vi "UI_Graph.vi"() -> ()   [LabVIEW 2016]
uses:
  PanelSplitToolkit/QueueManager.llb/Remove.vi
  PanelSplitToolkit/QueueManager.llb/Insert.vi
  PanelSplitToolkit/PanelRootNode/PanelRootNode.lvclass
  PCM PanelSplit/PCM PanelSplit.lvclass
  PanelSplitToolkit/QueueManager.llb/Destroy.vi
  <vilib>/Utility/error.llb/DialogType.ctl
  PanelSplitToolkit/QueueManager.llb/CreatQueue.vi
panel:
  in  "Caller":string
  in  "删除按钮":bool
  in  "添加按钮":bool
  in  "下一页":bool
  in  "上一页":bool
  in  "Page":u16(ring) items=["Page0"]
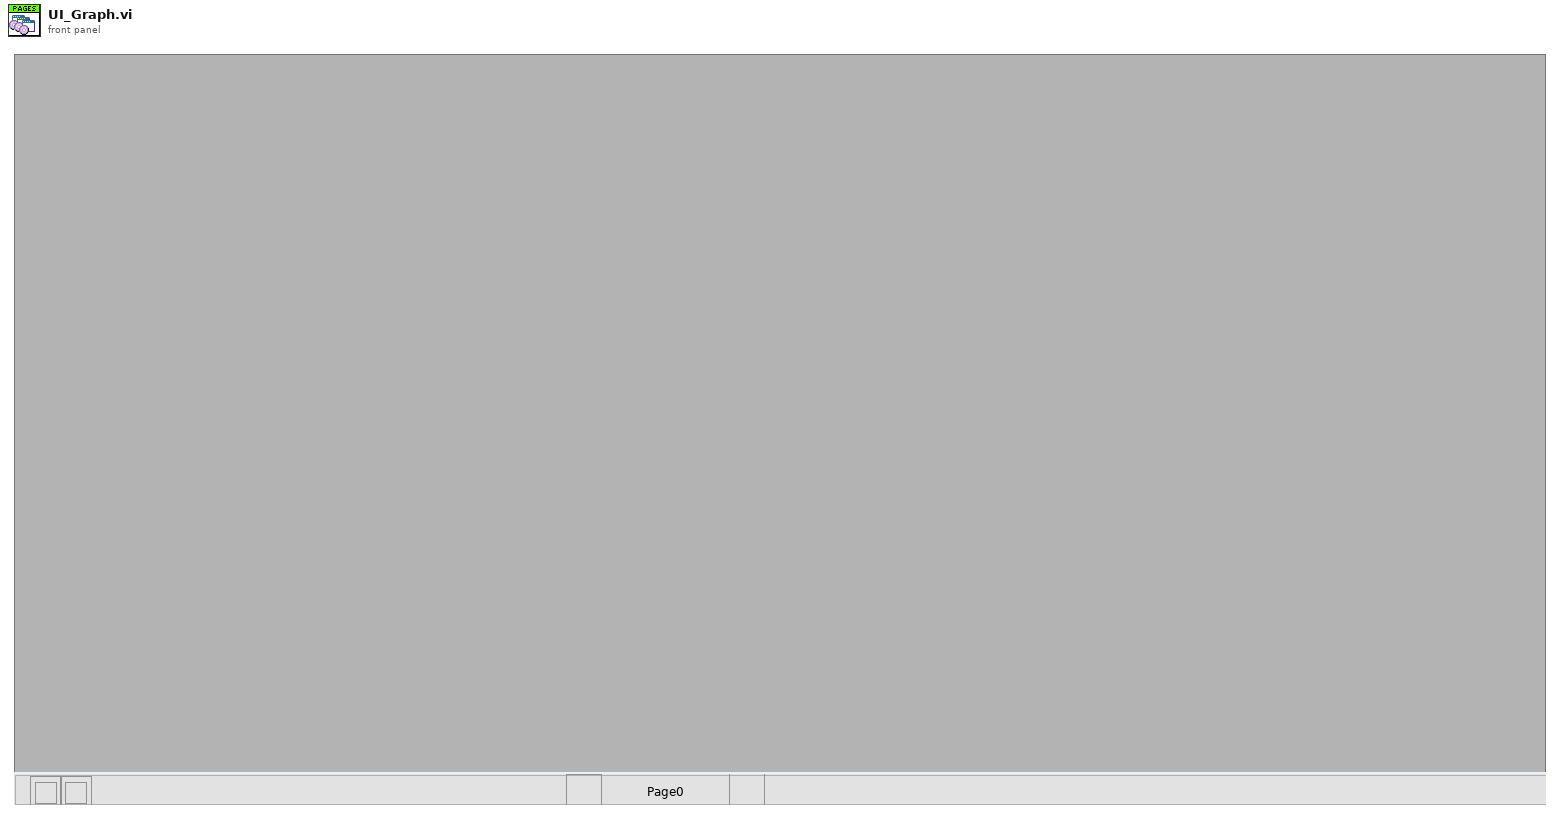
[diagram p1: front panel]
types:
  T1 = cluster{"error":errorcluster, "Event":string, "Data":variant, "Q_Local":string, "DyPageNames":string[], "DyPageVIRefs":refnum<vi>[], "PageTreeTags":string[], "CurrentPage":string, "PageVIPath":path, "PanelUIQName":string, "Send":cluster{"VI*ToSend":refnum<vi>, "EventToSend":string, "DataToSend":variant}, "PageCtr*":refnum<vi>, "SubPanel*":refnum<vi>, "Q_Caller":string, "FixedPages":cluster{"FixedPageNames":string[], "FixedPageVIRefs":refnum<vi>[]}}
  T2 = cluster{"Main Queue":string, "DAQ Queue":string, "ANA Queue":string, "CUI Queue":string, "Q-FocusList":string, "Q-Toolbar":string, "Q-Config":string}
  T3 = cluster{"Page":refnum<vi>, "SubPanel":refnum<vi>}
  T4 = typedef "DialogType.ctl" = u16
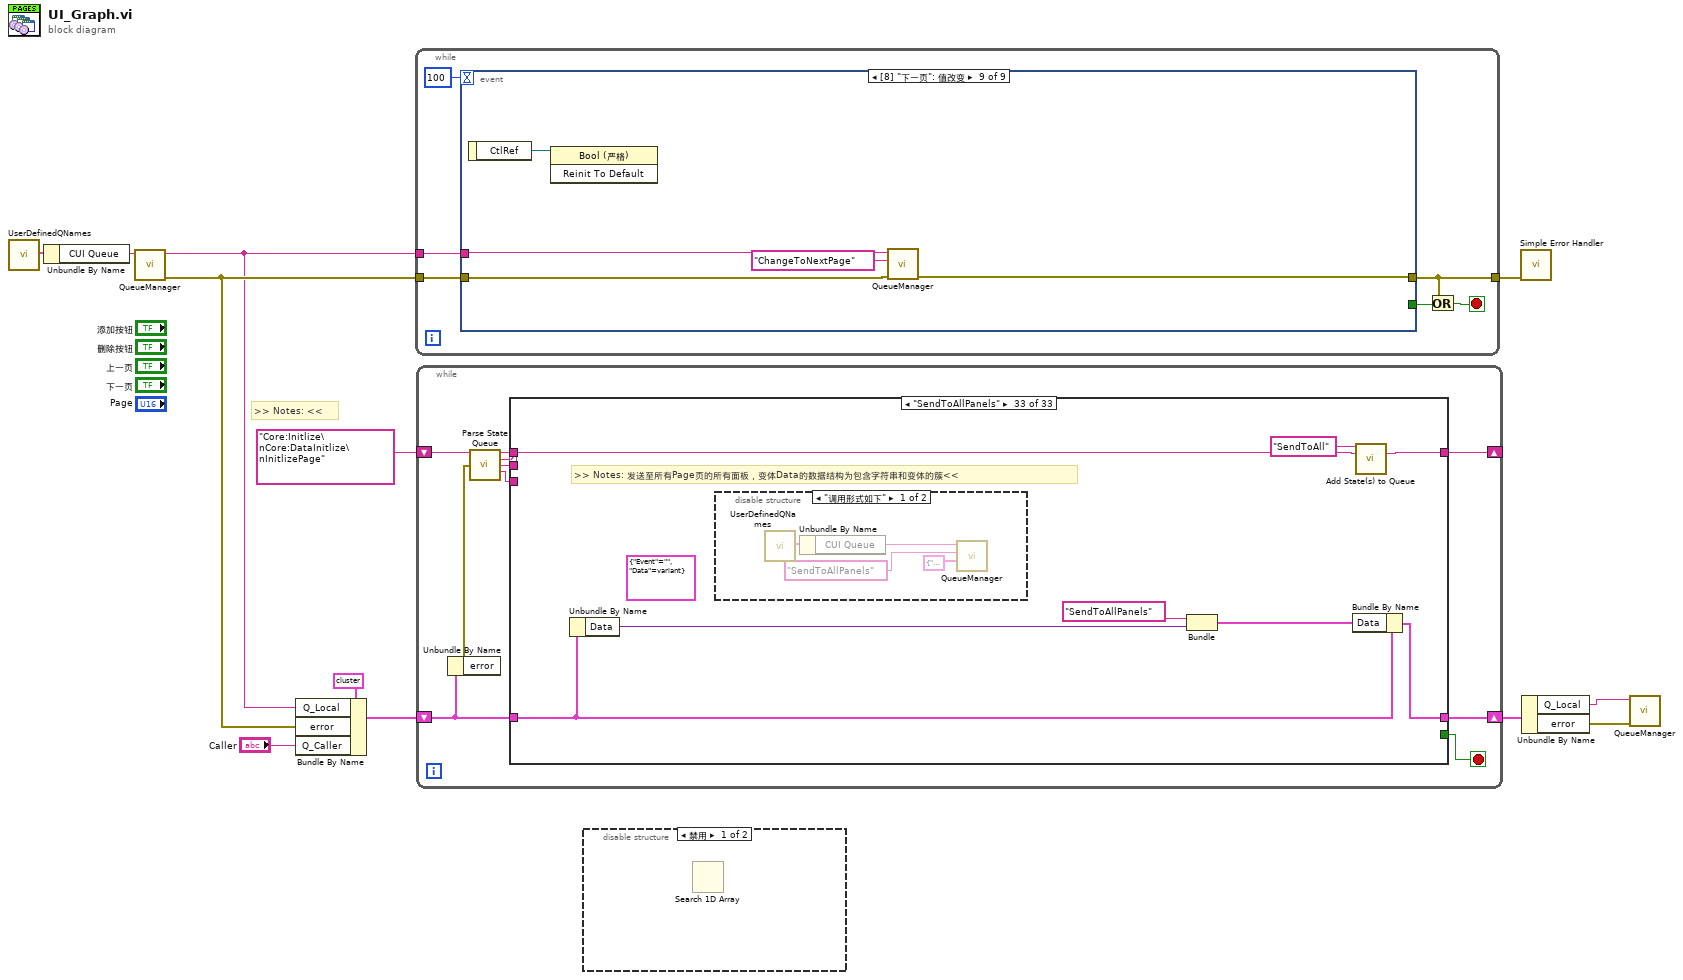
[diagram p0: block diagram]
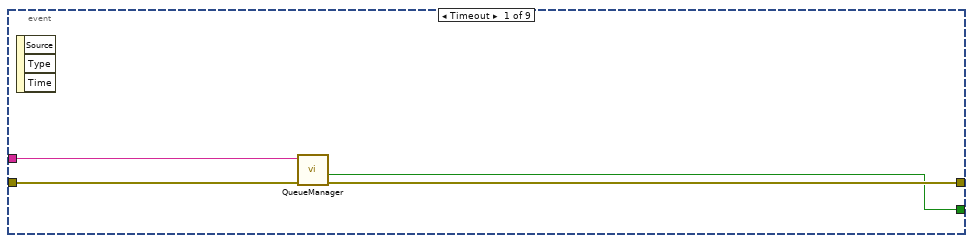
[diagram p2: hidden frame]
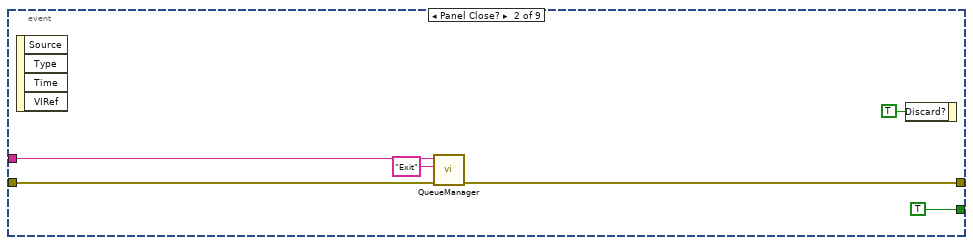
[diagram p3: hidden frame]
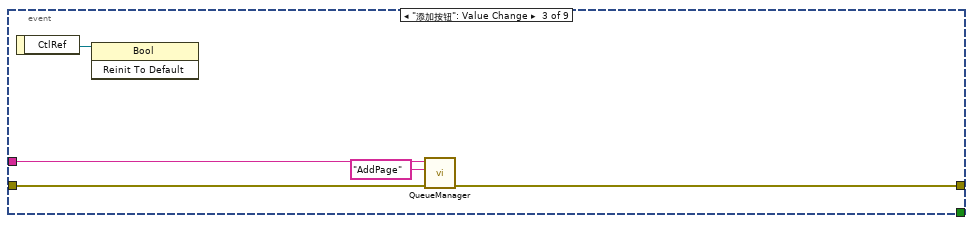
[diagram p4: hidden frame]
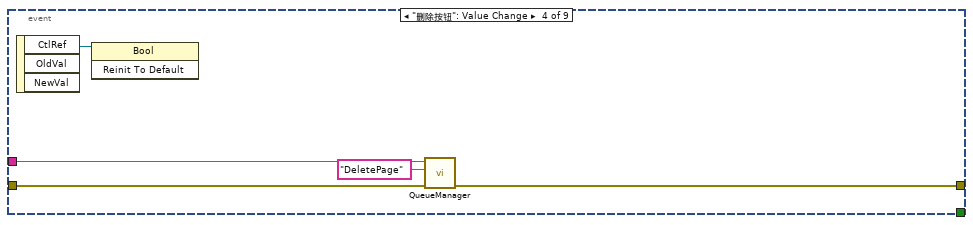
[diagram p5: hidden frame]
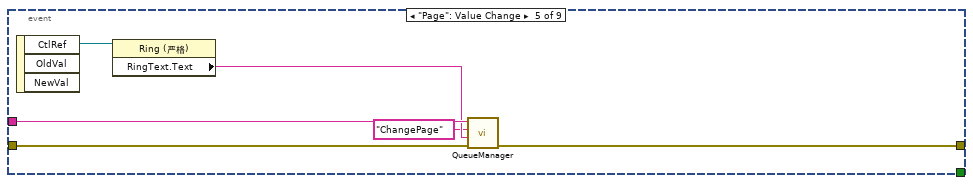
[diagram p6: hidden frame]
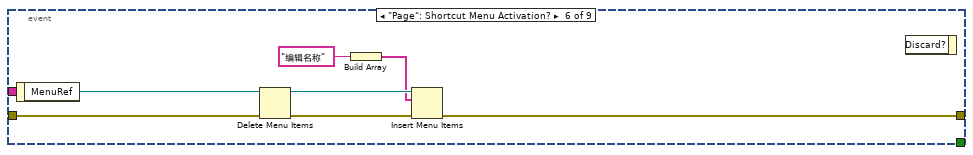
[diagram p7: hidden frame]
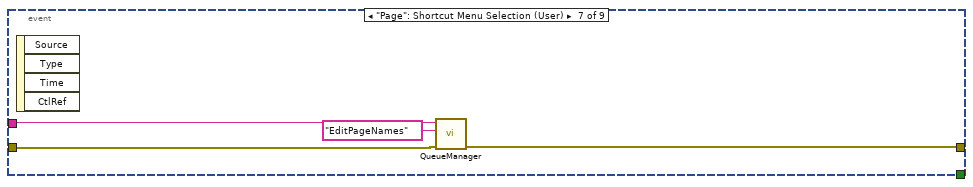
[diagram p8: hidden frame]
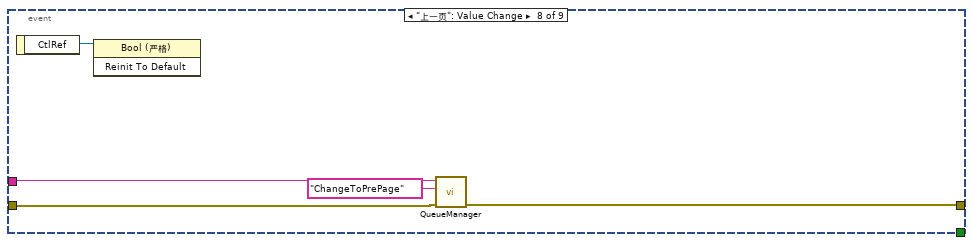
[diagram p9: hidden frame]
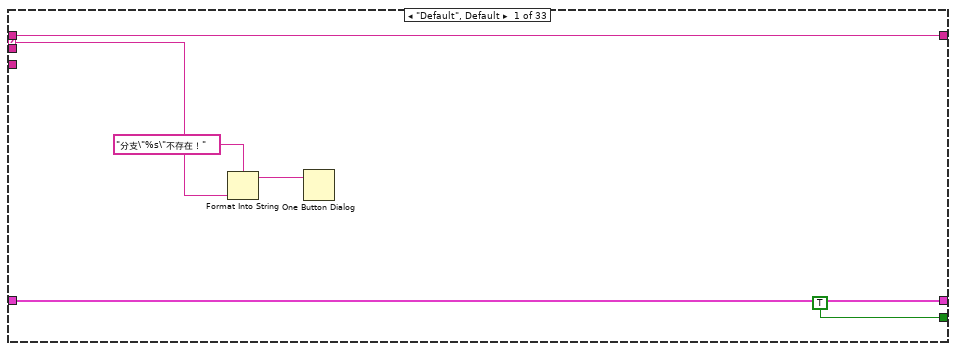
[diagram p11: hidden frame]
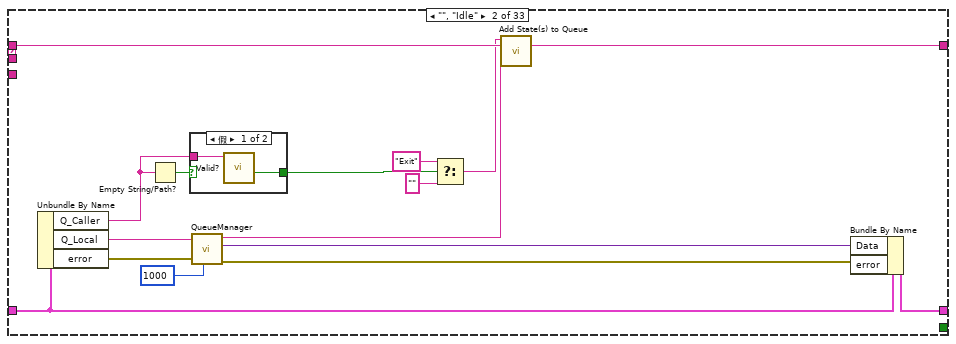
[diagram p12: hidden frame]
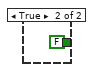
[diagram p13: hidden frame]
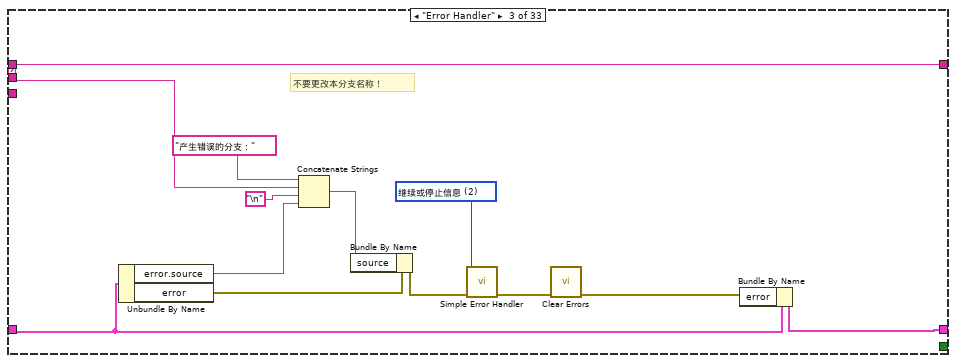
[diagram p14: hidden frame]
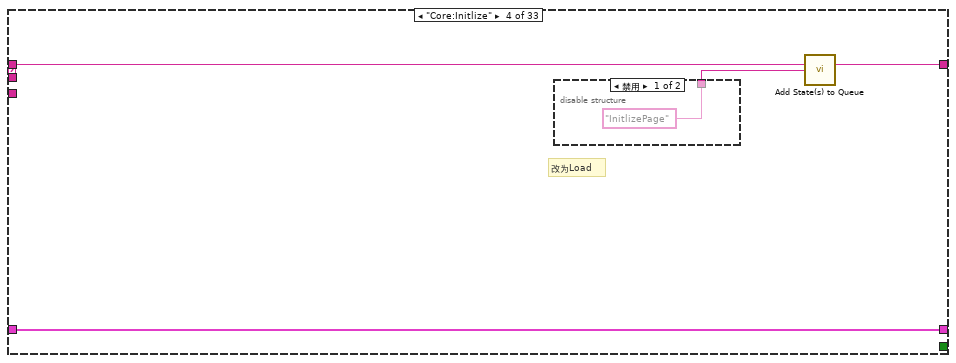
[diagram p15: hidden frame]
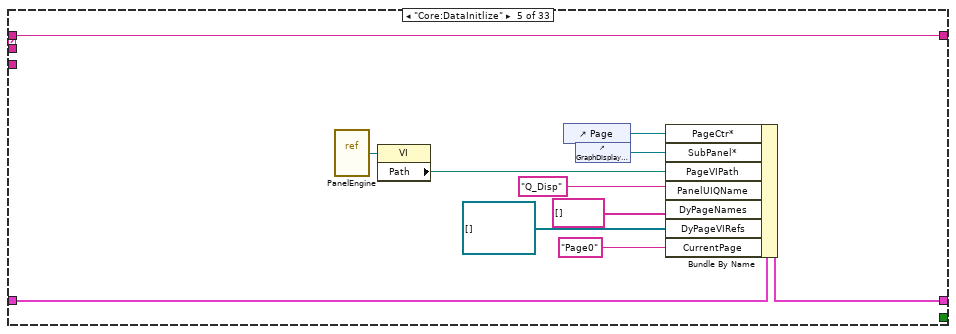
[diagram p17: hidden frame]
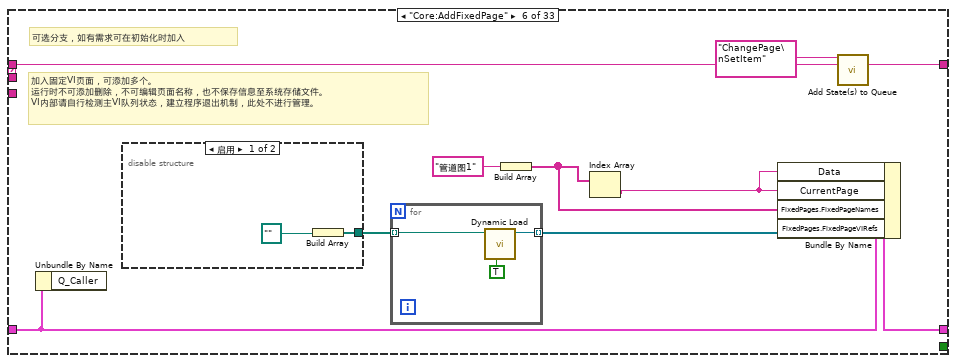
[diagram p18: hidden frame]
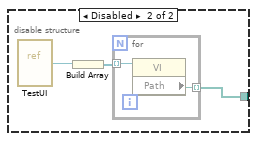
[diagram p19: hidden frame]
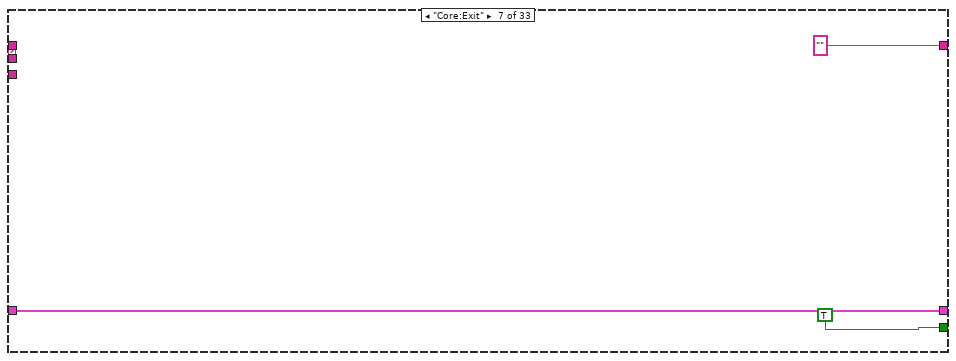
[diagram p20: hidden frame]
diagram:
  # ">> Notes: <<"
  n1 = call "UserDefinedQNames.vi"() -> ("All Queues"=w2:T2)  [unwired: 11 in]
  n2 = Unbundle By Name(w2) -> ("CUI Queue"=w1:string)
  n3 = call-poly "QueueManager.vi"("QueueName"=w1) -> ("error out"=w6:errorcluster, "QueueName out"=w4:string)  [unwired: 9 in]
  n4 = Bundle By Name(cluster=T1 {"error"={"status"=FALSE, "code"=0, "source"=""}, "Event"="", "Data"=variant, "Q_Local"="", "DyPageNames"=[], "DyPageVIRefs"=[], "PageTreeTags"=[], "CurrentPage"="", "PageVIPath"=path "", "PanelUIQName"="", "Send"={"VI*ToSend"=refnum, "EventToSend"="", "DataToSend"=variant}, "PageCtr*"=refnum, "SubPanel*"=refnum, "Q_Caller"="", "FixedPages"={"FixedPageNames"=[], "FixedPageVIRefs"=[]}} ("TmpData"), "Q_Local"=w4, "error"=w6, "Q_Caller"="Caller") -> (w8:T1)
  n5 = while {
    tunnel: w6 -> [w17]
    tunnel: [w15] -> w5
    tunnel: w4 -> [w13]
    stop <- w18 stop-if-true
    n6 = event shown="[8] \"下一页\": 值改变" {
      selector: _ -> [_ _ _ _ _ _ _ _ _]
      dyn-events: _ -> [_ _ _ _ _ _ _ _ _]
      timeout: 100 -> [_ _ _ _ _ _ _ _ _]
      tunnel: w17 -> [w21 w26 w31 w36 w42 w46 w55 w60 w65]
      tunnel: [w20 w25 w30 w35 w41 w45 w52 w57 w62] -> w15
      tunnel: [w19 TRUE _ _ _ _ _ _ _] -> w16
      tunnel: w13 -> [w22 w27 w32 w37 w43 _ w54 w59 w64]
      event Timeout {
        n7 = event-data() -> ()  [unwired: 1 in, 3 out]
        n8 = call-poly "QueueManager.vi"("error in (no error)"=w21, "Queue Name(unamed)"=w22) -> ("error out"=w20:errorcluster, "Not Exist?"=w19:bool)  [unwired: 8 in]
      }
      event Panel Close? {
        n9 = event-data() -> ()  [unwired: 1 in, 4 out]
        n10 = call-poly "QueueManager.vi"("error in"=w26, "Event"="Exit", "QueueName"=w27) -> ("error out"=w25:errorcluster)  [unwired: 7 in, 1 out]
        n11 = event-data("Discard?"=TRUE ("放弃？")) -> ()  [unwired: 1 in, 1 out]
      }
      event "添加按钮": Value Change {
        n12 = event-data() -> ("CtlRef"=w33:refnum<vi>)  [unwired: 1 in]
        n13 = invoke class="Bool" method="Reinit To Default"(reference=w33) -> ()  [unwired: 2 in, 3 out]
        n14 = call-poly "QueueManager.vi"("error in"=w31, "Event"="AddPage", "QueueName"=w32) -> ("error out"=w30:errorcluster)  [unwired: 7 in, 1 out]
      }
      event "删除按钮": Value Change {
        n15 = event-data() -> ("CtlRef"=w38:refnum<vi>)  [unwired: 1 in, 2 out]
        n16 = invoke class="Bool" method="Reinit To Default"(reference=w38) -> ()  [unwired: 2 in, 3 out]
        n17 = call-poly "QueueManager.vi"("error in"=w36, "Event"="DeletePage", "QueueName"=w37) -> ("error out"=w35:errorcluster)  [unwired: 7 in, 1 out]
      }
      event "Page": Value Change {
        n18 = event-data() -> ("CtlRef"=w44:refnum<vi>)  [unwired: 1 in, 2 out]
        n19 = property class="Ring (严格)"(reference=w44) -> ("RingText.Text"=w40:string)  [unwired: 1 in, 2 out]
        n20 = call-poly "QueueManager.vi"("error in"=w42, "Data"=w40, "Event"="ChangePage", "QueueName"=w43) -> ("error out"=w41:errorcluster)  [unwired: 6 in, 1 out]
      }
      event "Page": Shortcut Menu Activation? {
        n21 = event-data() -> ("MenuRef"=w47:refnum<k9>)  [unwired: 1 in]
        n22 = Delete Menu Items(6:w46, 9:w47) -> (0:w50:errorcluster, 3:w51:refnum<k9>)  [unwired: 2 in]
        n23 = Build Array("编辑名称") -> (w48:string[])
        n24 = Insert Menu Items(6:w50, 8:w48, 9:w51) -> (0:w45:errorcluster)  [unwired: 3 in, 2 out]
        n25 = event-data() -> ()  [unwired: 2 in, 1 out]
      }
      event "Page": Shortcut Menu Selection (User) {
        n26 = event-data() -> ()  [unwired: 1 in, 4 out]
        n27 = call-poly "QueueManager.vi"("error in"=w55, "Event"="EditPageNames", "QueueName"=w54) -> ("error out"=w52:errorcluster)  [unwired: 7 in, 1 out]
      }
      event "上一页": Value Change {
        n28 = event-data() -> ("CtlRef"=w56:refnum<vi>)  [unwired: 1 in]
        n29 = invoke class="Bool (严格)" method="Reinit To Default"(reference=w56) -> ()  [unwired: 2 in, 3 out]
        n30 = call-poly "QueueManager.vi"("error in"=w60, "Event"="ChangeToPrePage", "QueueName"=w59) -> ("error out"=w57:errorcluster)  [unwired: 7 in, 1 out]
      }
      event "下一页": Value Change {
        n31 = event-data() -> ("CtlRef"=w61:refnum<vi>)  [unwired: 1 in]
        n32 = invoke class="Bool (严格)" method="Reinit To Default"(reference=w61) -> ()  [unwired: 2 in, 3 out]
        n33 = call-poly "QueueManager.vi"("error in"=w65, "Event"="ChangeToNextPage", "QueueName"=w64) -> ("error out"=w62:errorcluster)  [unwired: 7 in, 1 out]
      }
    }
    n34 = Or(x=w15, y=w16) -> (x .or. y?=w18:bool)
  }
  n35 = while {
    shift-right: [w68] -> w10
    shift-left: w8 -> [w69]
    shift-right: [w67] -> _
    shift-left: "Core:Initlize\nCore:DataInitlize\nInitlizePage" -> [w75]
    stop <- w71 stop-if-true
    n36 = Unbundle By Name(w69) -> ("error"=w70:errorcluster)
    n37 = call "Parse State Queue.vi"("State Queue"=w75, "Error In (no error)"=w70) -> ("Remaining States"=w74:string, "Current State"=w73:string, "Arguments"=w72:string, "PreState"=w66:string)  [unwired: 10 in]
    n38 = case shown="\"SendToAllPanels\"" w73 {
      selector: w73 -> [w79 _ _ _ _ _ _ _ _ _ _ _ _ _ _ _ _ _ _ _ _ _ _ _ _ _ _ _ _ _ _ _ _]
      tunnel: w74 -> [w80 w93 w113 w116 w129 w133 _ _ w158 w166 w168 w194 w219 w242 w257 w276 w278 w283 w304 w332 w336 w345 w403 w408 w433 w446 w457 w468 w472 w493 w495 w507 w517]
      tunnel: w72 -> [_ _ w101 _ _ _ _ _ _ _ _ _ _ _ _ _ _ _ _ _ _ _ _ _ _ _ _ _ _ _ _ _ _]
      tunnel: [TRUE _ _ _ _ _ TRUE FALSE FALSE _ _ _ _ _ _ _ FALSE FALSE _ _ _ _ _ _ _ _ _ _ _ _ _ _ _] -> w71
      tunnel: w69 -> [w81 w90 w103 w117 w128 w131 w151 w154 w162 w165 w176 w192 w209 w240 w261 w277 w279 w284 w313 w327 w338 w347 w395 w410 w435 w445 w448 w459 w477 w488 w494 w498 w519]
      tunnel: [w81 w96 w102 w117 w127 w139 w151 w153 w161 w165 w175 w191 w207 w239 w260 w277 w279 w285 w311 w326 w337 w346 w394 w409 w434 w445 w447 w458 w473 w486 w494 w497 w514] -> w68
      tunnel: [w80 w92 w113 w115 w129 w132 "" ("Remaining States") "SendToAll\nCore:Exit" ("Remaining States") w159 w166 w167 w194 w218 w241 w256 w275 w278 w282 w303 w332 w335 w344 w403 w407 w432 w446 w457 w468 w471 w493 w495 w507 w516] -> w67
      tunnel: w66 -> [_ _ _ _ _ _ _ _ _ _ _ _ _ _ _ _ _ _ _ _ _ _ _ _ _ _ _ _ _ _ _ _ _]
      frame "Default", Default {
        n39 = Format Into String(format string="分支\"%s\"不存在！" ("格式字符串"), w79) -> (resulting string=w78:string)  [unwired: 2 in, 1 out]
        n40 = One Button Dialog(message=w78) -> ()  [unwired: 1 in, 1 out]
      }
      frame "", "Idle" {
        n41 = Unbundle By Name(w90) -> ("Q_Caller"=w83:string, "Q_Local"=w89:string, "error"=w88:errorcluster)
        n42 = Empty String/Path?(string/path=w83) -> (empty?=w87:bool)
        n43 = case shown="假" w87 {
          tunnel: [w99 FALSE ("Not Exist?")] -> w86
          tunnel: w83 -> [w98 _]
          frame False {
            n44 = call "Valid?.vi"("Queue Name(unamed)"=w98) -> ("Not Exist?"=w99:bool)  [unwired: 9 in, 1 out]
          }
          frame True {
          }
        }
        n45 = call-poly "QueueManager.vi"("Time out(-1)"=1000, "error in (no error)"=w88, "Queue Name"=w89) -> ("error out"=w97:errorcluster, "Data"=w95:variant, "Event"=w94:string)  [unwired: 5 in, 1 out]
        n46 = Select(t="Exit" ("Event"), s=w86, f="") -> (s? t:f=w82:string)
        n47 = call "Add State(s) to Queue.vi"("State(s) in Front (\"\")"=w82, "State(s) in (\"\")"=w93, "State(s) at Back (\"\")"=w94) -> ("States Out"=w92:string)  [unwired: 12 in]
        n48 = Bundle By Name(cluster=w90, "Data"=w95, "error"=w97) -> (w96:T1)
      }
      frame "Error Handler" {
        w110 = T4 2 items=["无对话框", "确定信息", "继续或停止信息", "确定信息＋警告", "继续/停止+警告"] ("type of dialog (OK msg:1)")
        # "不要更改本分支名称！"
        n49 = Unbundle By Name(w103) -> ("error.source"=w104:string, "error"=w106:errorcluster)
        n50 = Concatenate Strings("产生错误的分支：" ("字符串"), w101, "\n", w104) -> (w107:string)
        n51 = Bundle By Name(cluster=w106, "source"=w107) -> (w105:errorcluster)
        n52 = call <vilib>:"Simple Error Handler.vi"("type of dialog (OK msg:1)"=w110, "error in (no error)"=w105) -> ("error out"=w111:errorcluster)  [unwired: 3 in, 4 out]
        n53 = call <vilib>:"Clear Errors.vi"("error in (no error)"=w111) -> ("error out"=w112:errorcluster)  [unwired: 5 in, 1 out]
        n54 = Bundle By Name(cluster=w103, "error"=w112) -> (w102:T1)
      }
      frame "Core:Initlize" {
        # "改为Load"
        n55 = disable-structure shown="禁用" {
          disable-tunnel: ["InitlizePage" ("State(s) at Back (\"\")") _] -> w114
          frame Disabled {
          }
          frame Enabled {
          }
        }
        n56 = call "Add State(s) to Queue.vi"("State(s) in (\"\")"=w116, "State(s) at Back (\"\")"=w114) -> ("States Out"=w115:string)  [unwired: 13 in]
      }
      frame "Core:DataInitlize" {
        n57 = vi-ref "PanelEngine.vi"() -> (w125:refnum<vi>)
        n58 = property class="VI"(reference=w125) -> ("Path"=w124:path)  [unwired: 1 in, 2 out]
        n59 = control-ref of="Page"() -> (w120:refnum<vi>)
        n60 = control-ref of="GraphDisplayPanel"() -> (w119:refnum<vi>)
        n61 = Bundle By Name(cluster=w128, "PageCtr*"=w120, "SubPanel*"=w119, "PageVIPath"=w124, "PanelUIQName"="Q_Disp", "DyPageNames"=string[] [] ("PageNames"), "DyPageVIRefs"=refnum<vi>[] [] ("PageVIRefs"), "CurrentPage"="Page0") -> (w127:T1)
      }
      frame "Core:AddFixedPage" {
        # "可选分支，如有需求可在初始化时加入"
        # "加入固定VI页面，可添加多个。\n运行时不可添加删除，不可编辑页面名称，也不保存信息至系统存储文件。\nVI内部请自行检测主VI队列状态，建立程序退出机制，此处不进行管理。"
        n62 = Unbundle By Name(w131) -> ()  [unwired: 1 out]
        n63 = disable-structure shown="启用" {
          disable-tunnel: [w140 w144] -> w137
          frame Enabled {
            n64 = Build Array(path "" ("Vi Path")) -> (w140:path[])
          }
          frame Disabled {
            n65 = vi-ref "TestUI.vi"() -> (w142:refnum<vi>)
            n66 = Build Array(w142) -> (w143:refnum<vi>[])
            n67 = for {
              tunnel: w143 -> [w146] mode=indexing
              tunnel: [w145] -> w144 mode=indexing
              n68 = property class="VI"(reference=w146) -> ("Path"=w145:path)  [unwired: 1 in, 2 out]
            }
          }
        }
        n69 = for {
          tunnel: [w149] -> w138 mode=indexing
          tunnel: w137 -> [w148] mode=indexing
          n70 = call "Dynamic Load.vi"("Auto Dispose Ref"=TRUE, "Vi Path"=w148) -> ("vi reference"=w149:refnum<vi>)  [unwired: 8 in, 1 out]
        }
        n71 = Build Array("管道图1") -> (w135:string[])
        n72 = Index Array(array=w135) -> (element=w130:string)  [unwired: 1 in]
        n73 = Bundle By Name(cluster=w131, "Data"=w130, "CurrentPage"=w130, "FixedPages.FixedPageNames"=w135, "FixedPages.FixedPageVIRefs"=w138) -> (w139:T1)
        n74 = call "Add State(s) to Queue.vi"("State(s) in Front (\"\")"="ChangePage\nSetItem" ("State(s) in Front (\"\")"), "State(s) in (\"\")"=w133) -> ("States Out"=w132:string)  [unwired: 13 in]
      }
      frame "Core:Exit" {
      }
      frame "Exit" {
        n75 = Bundle By Name(cluster=w154, "Data"=cluster{string, "变体":variant} {"Exit", "变体"=variant}) -> (w153:T1)
      }
      frame "Clear" {
        n76 = Bundle By Name(cluster=w162, "Data"=cluster{string, "变体":variant} {"Exit", "变体"=variant}) -> (w161:T1)
        n77 = call "Add State(s) to Queue.vi"("State(s) in Front (\"\")"="SendToAll\nCore:DataInitlize" ("Remaining States"), "State(s) in (\"\")"=w158) -> ("States Out"=w159:string)  [unwired: 13 in]
      }
      frame "--------Init------------" {
      }
      frame "Initlize" {
        n78 = Unbundle By Name(w176) -> ("Data"=w178:variant, "error"=w170:errorcluster)
        n79 = Variant To Data(error in=w170, type=T3 {"Page"=refnum, "SubPanel"=refnum}, Variant=w178) -> (data=w174:T3, error out=w171:errorcluster)
        n80 = Unbundle By Name(w174) -> ("Page"=w173:refnum<vi>, "SubPanel"=w172:refnum<vi>)
        n81 = Bundle By Name(cluster=w176, "PageCtr*"=w173, "SubPanel*"=w172, "error"=w171) -> (w175:T1)
        n82 = call "Add State(s) to Queue.vi"("State(s) in (\"\")"=w168, "State(s) at Back (\"\")"="InitlizePage" ("State(s) in Front (\"\")")) -> ("States Out"=w167:string)  [unwired: 13 in]
      }
      frame "Save" {
        w189 = ""  # Q_Name
        # ">> Notes: 获取所有Page页的保存信息，发送给请求保存的队列<<"
        n83 = Unbundle By Name(w192) -> ("DyPageNames"=w180:string[], "DyPageVIRefs"=w193:refnum<vi>[], "Data"=w190:variant, "error"=w183:errorcluster)
        n84 = Variant To Data(error in=w183, type=w189, Variant=w190) -> (data=w186:string, error out=w184:errorcluster)
        n85 = for {
          tunnel: w193 -> [w198] mode=indexing
          tunnel: [w200] -> w182 mode=indexing
          shift-right: [w199] -> w188
          shift-left: w184 -> [w195]
          n86 = call "Get RootNodebyVIRef.vi"("error in"=w195, "vi*"=w198) -> ("error out"=w196:errorcluster, "RootNode*"=w197:refnum<data-value>)  [unwired: 8 in]
          n87 = in-place {
            in-place-border: w196 -> [w203]
            in-place-border: [w202] -> w199
            in-place-border: [w201] -> w200
            n88 = in-place-dvr #1(w197) -> (w205:refnum<class "PanelRootNode.lvclass">)  [unwired: 1 out]
            n89 = call-dynamic "GetXmlString.vi"("error in"=w203, "PanelRootNode 输入"=w205) -> ("error out"=w202:errorcluster, "XML"=w201:string, "PanelRootNode 输出"=w204:refnum<class "PanelRootNode.lvclass">)  [unwired: 7 in]
            n90 = in-place-dvr #1(w204) -> ()  [unwired: 2 out]
          }
        }
        n91 = Flatten To XML(anything=w180) -> (xml string=w179:string)
        n92 = Build Array (concatenate)(w179, w182) -> (w181:string[])
        n93 = call-poly "QueueManager.vi"("error in"=w188, "Data"=w181, "Event"="Save", "QueueName"=w186) -> ("error out"=w187:errorcluster)  [unwired: 6 in, 1 out]
        n94 = Bundle By Name(cluster=w192, "error"=w187) -> (w191:T1)
      }
      frame "Load11" {
        # ">> Notes: 装载配置信息\n1.清除当前所有图和页面\n2.根据配置信息增加相应页\n3.每个页读取配置文件进行分割及节点赋值<<"
        n95 = Unbundle By Name(w209) -> ("Q_Local"=w211:string, "Data"=w216:variant)
        n96 = call-poly "QueueManager.vi"("Event"="Clear", "QueueName"=w211) -> ("error out"=w214:errorcluster)  [unwired: 8 in, 1 out]
        n97 = Variant To Data(error in=w214, type=string[] [], Variant=w216) -> (data=w206:string[], error out=w213:errorcluster)
        n98 = for {
          tunnel: w211 -> [w222]
          tunnel: w206 -> [_] mode=indexing
          shift-right: [w220] -> w212
          shift-left: w213 -> [w223]
          n99 = call-poly "QueueManager.vi"("error in"=w223, "Event"="AddPage", "QueueName"=w222) -> ("error out"=w220:errorcluster)  [unwired: 7 in, 1 out]
        }
        n100 = call-poly "QueueManager.vi"("error in"=w212, "Data"=w206, "Event"="LoadXml", "QueueName"=w211) -> ("error out"=w208:errorcluster)  [unwired: 6 in, 1 out]
        n101 = call "Add State(s) to Queue.vi"("State(s) in (\"\")"=w219) -> ("States Out"=w218:string)  [unwired: 14 in]
        n102 = Bundle By Name(cluster=w209, "error"=w208) -> (w207:T1)
      }
      frame "Load" {
        # ">> Notes: 装载配置信息\n1.清除当前所有图和页面\n2.根据配置信息增加相应页\n3.每个页读取配置文件进行分割及节点赋值<<"
        n103 = Unbundle By Name(w240) -> ("SubPanel*"=w231:refnum<vi>, "PageVIPath"=w232:path, "Data"=w235:variant, "DyPageVIRefs"=w238:refnum<vi>[], "error"=w237:errorcluster, "FixedPages.FixedPageNames"=w226:string[])
        n104 = for {
          tunnel: w238 -> [w250] mode=indexing
          shift-right: [w248] -> w236
          shift-left: w237 -> [w247]
          n105 = call "GetViName.vi"("VI*"=w250) -> ("VI Name"=w249:string)  [unwired: 9 in, 1 out]
          n106 = call-poly "QueueManager.vi"("error in"=w247, "Event"="Exit", "QueueName"=w249) -> ("error out"=w248:errorcluster)  [unwired: 7 in, 1 out]
        }
        n107 = Index Array(array=w226) -> (element=w225:string)  [unwired: 1 in]
        n108 = Variant To Data(error in=w236, Variant=w235) -> (data=w233:string[], error out=w234:errorcluster)  [unwired: 1 in]
        n109 = call "PageLoad.vi"("error in"=w234, "SubPanel*"=w231, "PanelVIPath"=w232, "data"=w233) -> ("error out"=w224:errorcluster, "PageNames"=w229:string[], "VIRefs"=w230:refnum<vi>[])  [unwired: 5 in]
        n110 = disable-structure shown="启用" {
          disable-tunnel: w229 -> [w244 _]
          disable-tunnel: [w243 w245] -> w228
          disable-tunnel: w225 -> [_ w245]
          frame Enabled {
            n111 = Index Array(array=w244) -> (element=w243:string)  [unwired: 1 in]
          }
          frame Disabled {
          }
        }
        n112 = call "Add State(s) to Queue.vi"("State(s) in Front (\"\")"="ChangePage\nSetItem" ("State(s) in Front (\"\")"), "State(s) in (\"\")"=w242) -> ("States Out"=w241:string)  [unwired: 13 in]
        n113 = Bundle By Name(cluster=w240, "DyPageVIRefs"=w230, "DyPageNames"=w229, "error"=w224, "Data"=w228) -> (w239:T1)
      }
      frame "LoadXml" {
        n114 = Unbundle By Name(w261) -> ("DyPageVIRefs"=w262:refnum<vi>[], "Data"=w255:variant, "error"=w251:errorcluster)
        n115 = Variant To Data(error in=w251, type=string[] [], Variant=w255) -> (data=w254:string[], error out=w252:errorcluster)
        n116 = for {
          tunnel: w262 -> [w273] mode=indexing
          tunnel: w254 -> [w272] mode=indexing
          tunnel: [w269] -> w259 mode=indexing
          tunnel: w252 -> [w263]
          n117 = call "GetViName.vi"("VI*"=w273) -> ("VI Name"=w268:string)  [unwired: 9 in, 1 out]
          n118 = call-poly "QueueManager.vi"("error in"=w263, "Data"=w272, "Event"="LoadXmlString", "QueueName"=w268) -> ("error out"=w270:errorcluster)  [unwired: 6 in, 1 out]
          n119 = Bundle By Name(cluster=cluster{"Event":string, "Data":variant} {"Event"="", "Data"=variant} ("Send"), "Event"="Load") -> (w265:cluster{"Event":string, "Data":variant})
          n120 = call-poly "QueueManager.vi"("error in"=w270, "Data"=w265, "Event"="SendToAllPanels", "QueueName"=w268) -> ("error out"=w269:errorcluster)  [unwired: 6 in, 1 out]
        }
        n121 = Merge Errors(w259) -> (w258:errorcluster)
        n122 = call "Add State(s) to Queue.vi"("State(s) in (\"\")"=w257) -> ("States Out"=w256:string)  [unwired: 14 in]
        n123 = Bundle By Name(cluster=w261, "error"=w258) -> (w260:T1)
      }
      frame "New" {
        # ">> Notes: 响应主程序的“新建”指令，清除所有页面，然后加载一个波形图表<<"
        n124 = call "Add State(s) to Queue.vi"("State(s) in (\"\")"=w276, "State(s) at Back (\"\")"="Clear\nAddPage" ("State(s) at Back (\"\")")) -> ("States Out"=w275:string)  [unwired: 13 in]
      }
      frame "-----PageManager------" {
      }
      frame "InitlizePage" {
        n125 = disable-structure shown="启用" {
          disable-tunnel: [w297 w298] -> w285
          disable-tunnel: w284 -> [w296 w298]
          disable-tunnel: ["ChangePage" ("State(s) in Front (\"\")") "AddPage" ("State(s) in Front (\"\")")] -> w281
          frame Disabled {
            w289 = "Page0" ("CurrentPage")
            n126 = Unbundle By Name(w296) -> ("PageVIPath"=w295:path, "error"=w293:errorcluster)
            n127 = call "Dynamic Load.vi"("Auto Dispose Ref"=TRUE ("自动销毁引用"), "error in"=w293, "Vi Path"=w295) -> ("错误输出"=w290:errorcluster, "vi reference"=w294:refnum<vi>)  [unwired: 7 in]
            n128 = Build Array(w294) -> (w292:refnum<vi>[])
            n129 = Build Array(w289) -> (w291:string[])
            n130 = Bundle By Name(cluster=w296, "CurrentPage"=w289, "DyPageNames"=w291, "DyPageVIRefs"=w292, "error"=w290, "Data"=w289) -> (w297:T1)
          }
          frame Enabled {
          }
        }
        n131 = call "Add State(s) to Queue.vi"("State(s) in Front (\"\")"=w281, "State(s) in (\"\")"=w283) -> ("States Out"=w282:string)  [unwired: 13 in]
      }
      frame "AddPage" {
        n132 = Unbundle By Name(w313) -> ("DyPageVIRefs"=w309:refnum<vi>[], "PageVIPath"=w310:path, "DyPageNames"=w301:string[])
        n133 = for {
          N: 100 -> [_]
          tunnel: w301 -> [w319]
          tunnel: "Page" -> [w322]
          tunnel: [w316] -> w305
          i -> [w321]
          stop <- w317 stop-if-true
          n134 = Number To Decimal String(number=w321) -> (decimal integer string=w320:string)  [unwired: 1 in]
          n135 = Concatenate Strings(w322, w320) -> (w316:string)
          n136 = Search 1D Array(1D array=w319, element=w316) -> (index of element=w318:i32)  [unwired: 1 in]
          n137 = Less Than 0?(x=w318) -> (x < 0?=w317:bool)
        }
        n138 = call "Dynamic Load.vi"("Auto Dispose Ref"=TRUE ("自动销毁引用"), "Vi Path"=w310) -> ("错误输出"=w307:errorcluster, "vi reference"=w308:refnum<vi>)  [unwired: 8 in]
        n139 = Build Array (concatenate)(w301, w305) -> (w312:string[])
        n140 = Build Array (concatenate)(w309, w308) -> (w306:refnum<vi>[])
        n141 = Bundle By Name(cluster=w313, "DyPageVIRefs"=w306, "error"=w307, "DyPageNames"=w312, "Data"=w305) -> (w311:T1)
        n142 = call "Add State(s) to Queue.vi"("State(s) in Front (\"\")"="ChangePage\nSetItem" ("State(s) in Front (\"\")"), "State(s) in (\"\")"=w304) -> ("States Out"=w303:string)  [unwired: 13 in]
      }
      frame "SetItem" {
        n143 = Unbundle By Name(w327) -> ("FixedPages.FixedPageNames"=w325:string[], "DyPageNames"=w324:string[], "PageCtr*"=w331:refnum<vi>, "CurrentPage"=w330:string)
        n144 = Build Array (concatenate)(w325, w324) -> (w323:string[])
        n145 = Search 1D Array(1D array=w323, element=w330) -> (index of element=w329:i32)  [unwired: 1 in]
        n146 = property class="Ring"(reference=w331, "Strings []"=w323, "Value"=w329) -> (error out=w328:errorcluster)  [unwired: 1 in, 1 out]
        n147 = Bundle By Name(cluster=w327, "error"=w328) -> (w326:T1)
      }
      frame "EditPageNames" {
        n148 = Unbundle By Name(w338) -> ("DyPageNames"=w334:string[], "PageCtr*"=w340:refnum<vi>)
        n149 = call "EditPageNames UI.vi"("PageNames"=w334) -> ("PageNames out"=w333:string[])  [unwired: 10 in]
        n150 = property class="Ring"(reference=w340, "Strings []"=w333) -> (error out=w339:errorcluster)  [unwired: 1 in, 1 out]
        n151 = Bundle By Name(cluster=w338, "DyPageNames"=w333, "error"=w339) -> (w337:T1)
        n152 = call "Add State(s) to Queue.vi"("State(s) in (\"\")"=w336) -> ("States Out"=w335:string)  [unwired: 14 in]
      }
      frame "DeletePage" {
        n153 = Unbundle By Name(w347) -> ("DyPageVIRefs"=w348:refnum<vi>[], "DyPageNames"=w343:string[], "CurrentPage"=w342:string)
        n154 = Search 1D Array(1D array=w343, element=w342) -> (index of element=w341:i32)  [unwired: 1 in]
        n155 = case shown="0, 默认" w341 {
          tunnel: w348 -> [_ w365]
          tunnel: w347 -> [w351 w364]
          tunnel: [w351 w361] -> w346
          tunnel: w345 -> [w350 w359]
          tunnel: [w350 w358] -> w344
          tunnel: w343 -> [_ w353]
          tunnel: w342 -> [_ w352]
          frame -1 {
            n156 = One Button Dialog(message="该页面不允许删除！" ("消息")) -> ()  [unwired: 1 in, 1 out]
          }
          frame 0, Default {
            n157 = Array Size(array=w353) -> (size(s)=w360:i32)
            n158 = case shown="2.., 默认" w360 {
              tunnel: w352 -> [w379 w382]
              tunnel: w365 -> [w377 w384]
              tunnel: [w373 w385] -> w363
              tunnel: [w375 w384] -> w362
              tunnel: w353 -> [w374 w385]
              tunnel: [w372 w382] -> w357
              tunnel: ["ChangePage\nSendToSingle\nSetItem" ("State(s) in Front (\"\")") "" ("State(s) in Front (\"\")")] -> w356
              tunnel: [w367 refnum<vi> refnum ("VI引用")] -> w355
              tunnel: ["Exit" ""] -> w354
              frame 2.., Default {
                # "删除页名、VI引用，切换到页面、关闭删除的VI、删除控件对应项"
                # "切换到第0页"
                n159 = Search 1D Array(1D array=w374, element=w379) -> (index of element=w370:i32)  [unwired: 1 in]
                n160 = Delete From Array(array=w374, length=1 ("长度"), index=w370) -> (array with subset deleted=w373:string[])  [unwired: 1 out]
                n161 = Delete From Array(array=w377, length=1 ("长度"), index=w370) -> (deleted portion=w368:refnum<vi>[], array with subset deleted=w375:refnum<vi>[])
                n162 = Index Array(array=w368) -> (element=w367:refnum<vi>)  [unwired: 1 in]
                n163 = Index Array(array=w373, index=0 ("索引")) -> (element=w372:string)
              }
              frame 1 {
                # "只有一页时不允许删"
              }
            }
            n164 = Bundle By Name(cluster=w364, "DyPageNames"=w363, "DyPageVIRefs"=w362, "Data"=w357, "Send.VI*ToSend"=w355, "Send.EventToSend"=w354) -> (w361:T1)
            n165 = call "Add State(s) to Queue.vi"("State(s) in Front (\"\")"=w356, "State(s) in (\"\")"=w359) -> ("States Out"=w358:string)  [unwired: 13 in]
          }
        }
      }
      frame "ChangePage" {
        n166 = Unbundle By Name(w395) -> ("SubPanel*"=w392:refnum<vi>, "FixedPages.FixedPageVIRefs"=w388:refnum<vi>[], "DyPageVIRefs"=w387:refnum<vi>[], "FixedPages.FixedPageNames"=w391:string[], "DyPageNames"=w390:string[], "Data"=w402:variant, "error"=w401:errorcluster)
        n167 = Variant To Data(error in=w401, type="" ("PageName"), Variant=w402) -> (data=w393:string, error out=w397:errorcluster)
        n168 = Build Array (concatenate)(w388, w387) -> (w386:refnum<vi>[])
        n169 = Build Array (concatenate)(w391, w390) -> (w389:string[])
        n170 = Search 1D Array(1D array=w389, element=w393) -> (index of element=w399:i32)  [unwired: 1 in]
        n171 = Index Array(array=w386, index=w399) -> (element=w398:refnum<vi>)
        n172 = invoke class="SubPnl" method="Insert VI"(reference=w392, error in=w397, "VI Ref"=w398) -> (error out=w396:errorcluster)  [unwired: 1 in, 3 out]
        n173 = Bundle By Name(cluster=w395, "error"=w396, "CurrentPage"=w393) -> (w394:T1)
      }
      frame "ChangeToPrePage" {
        n174 = Unbundle By Name(w410) -> ("PageCtr*"=w423:refnum<vi>, "error"=w412:errorcluster)
        n175 = property class="Ring"(reference=w423, error in=w412) -> (reference out=w415:refnum<vi>, error out=w414:errorcluster, "Strings []"=w418:string[], "RingText.Text"=w422:string)
        n176 = Array Size(array=w418) -> (size(s)=w417:i32)
        n177 = Search 1D Array(1D array=w418, element=w422) -> (index of element=w421:i32)  [unwired: 1 in]
        n178 = Equal To 0?(x=w421) -> (x = 0?=w420:bool)
        n179 = Decrement(x=w417) -> (x-1=w416:i32)
        n180 = Decrement(x=w421) -> (x-1=w419:i32)
        n181 = Select(t=w416, s=w420, f=w419) -> (s? t:f=w413:i32)
        n182 = To Unsigned Word Integer(number=w413) -> (unsigned 16bit integer=w405:u16)
        n183 = property class="Ring"(reference=w415, error in=w414, "Value"=w405) -> (error out=w411:errorcluster, "RingText.Text"=w404:string)  [unwired: 1 out]
        n184 = Bundle By Name(cluster=w410, "error"=w411, "Data"=w404) -> (w409:T1)
        n185 = call "Add State(s) to Queue.vi"("State(s) in Front (\"\")"="ChangePage" ("State(s) in Front (\"\")"), "State(s) in (\"\")"=w408) -> ("States Out"=w407:string)  [unwired: 13 in]
      }
      frame "ChangeToNextPage" {
        n186 = Unbundle By Name(w435) -> ("PageCtr*"=w444:refnum<vi>, "error"=w437:errorcluster)
        n187 = property class="Ring"(reference=w444, error in=w437) -> (reference out=w439:refnum<vi>, error out=w438:errorcluster, "Strings []"=w441:string[], "RingText.Text"=w443:string)
        n188 = Array Size(array=w441) -> (size(s)=w440:i32)
        n189 = Search 1D Array(1D array=w441, element=w443) -> (index of element=w430:i32)  [unwired: 1 in]
        n190 = Decrement(x=w440) -> (x-1=w429:i32)
        n191 = Increment(x=w430) -> (x+1=w442:i32)
        n192 = Equal?(x=w429, y=w430) -> (x = y?=w428:bool)
        n193 = Select(t=0, s=w428, f=w442) -> (s? t:f=w426:i32)
        n194 = To Unsigned Word Integer(number=w426) -> (unsigned 16bit integer=w425:u16)
        n195 = property class="Ring"(reference=w439, error in=w438, "Value"=w425) -> (error out=w436:errorcluster, "RingText.Text"=w424:string)  [unwired: 1 out]
        n196 = Bundle By Name(cluster=w435, "error"=w436, "Data"=w424) -> (w434:T1)
        n197 = call "Add State(s) to Queue.vi"("State(s) in Front (\"\")"="ChangePage" ("State(s) in Front (\"\")"), "State(s) in (\"\")"=w433) -> ("States Out"=w432:string)  [unwired: 13 in]
      }
      frame "-----PanelManager------" {
      }
      frame "AddPanel" {
        n198 = Unbundle By Name(w448) -> ("DyPageVIRefs"=w454:refnum<vi>[], "DyPageNames"=w455:string[], "CurrentPage"=w456:string)
        n199 = Search 1D Array(1D array=w455, element=w456) -> (index of element=w453:i32)  [unwired: 1 in]
        n200 = Index Array(array=w454, index=w453) -> (element=w452:refnum<vi>)
        n201 = call "GetViName.vi"("VI*"=w452) -> ("VI Name"=w451:string)  [unwired: 9 in, 1 out]
        n202 = call-poly "QueueManager.vi"("Event"="AddPanel", "QueueName"=w451) -> ("error out"=w449:errorcluster)  [unwired: 8 in, 1 out]
        n203 = Bundle By Name(cluster=w448, "error"=w449) -> (w447:T1)
      }
      frame "DeletePanel" {
        n204 = Unbundle By Name(w459) -> ("DyPageVIRefs"=w465:refnum<vi>[], "DyPageNames"=w466:string[], "CurrentPage"=w467:string)
        n205 = Search 1D Array(1D array=w466, element=w467) -> (index of element=w464:i32)  [unwired: 1 in]
        n206 = Index Array(array=w465, index=w464) -> (element=w463:refnum<vi>)
        n207 = call "GetViName.vi"("VI*"=w463) -> ("VI Name"=w462:string)  [unwired: 9 in, 1 out]
        n208 = call-poly "QueueManager.vi"("Event"="DeletePanel", "QueueName"=w462) -> ("error out"=w460:errorcluster)  [unwired: 8 in, 1 out]
        n209 = Bundle By Name(cluster=w459, "error"=w460) -> (w458:T1)
      }
      frame "TransferToSingle" {
        # "转发给当前PAGE的Panel引擎"
        n210 = Unbundle By Name(w477) -> ("DyPageVIRefs"=w479:refnum<vi>[], "DyPageNames"=w480:string[], "CurrentPage"=w481:string)
        n211 = Unbundle By Name(w477) -> ("Data"=w484:variant)
        n212 = Variant To Data(type=cluster{"Event":string, "Data":variant} {"Event"="", "Data"=variant}, Variant=w484) -> (data=w482:cluster{"Event":string, "Data":variant}, error out=w469:errorcluster)  [unwired: 1 in]
        n213 = Search 1D Array(1D array=w480, element=w481) -> (index of element=w478:i32)  [unwired: 1 in]
        n214 = Unbundle By Name(w482) -> ("Event"=w475:string, "Data"=w476:variant)
        n215 = Index Array(array=w479, index=w478) -> (element=w474:refnum<vi>)
        n216 = Bundle By Name(cluster=w477, "Send.VI*ToSend"=w474, "Send.EventToSend"=w475, "Send.DataToSend"=w476, "error"=w469) -> (w473:T1)
        n217 = call "Add State(s) to Queue.vi"("State(s) in Front (\"\")"="SendToSingle" ("State(s) in Front (\"\")"), "State(s) in (\"\")"=w472) -> ("States Out"=w471:string)  [unwired: 13 in]
      }
      frame "SendToSingle" {
        n218 = Unbundle By Name(w488) -> ("Send.EventToSend"=w489:string, "Send.DataToSend"=w490:variant, "Send.VI*ToSend"=w491:refnum<vi>, "error"=w485:errorcluster)
        n219 = call "GetViName.vi"("VI*"=w491) -> ("VI Name"=w492:string)  [unwired: 9 in, 1 out]
        n220 = call-poly "QueueManager.vi"("error in"=w485, "Data"=w490, "Event"=w489, "QueueName"=w492) -> ("error out"=w487:errorcluster)  [unwired: 6 in, 1 out]
        n221 = Bundle By Name(cluster=w488, "error"=w487) -> (w486:T1)
      }
      frame "--------Send----------" {
      }
      frame "SendToAll" {
        # ">> Notes: 发送给所有PanelEngine，不是发送给所有叶子节点面板<<"
        n222 = Unbundle By Name(w498) -> ("DyPageVIRefs"=w506:refnum<vi>[], "Data"=w505:variant, "error"=w500:errorcluster)
        n223 = Variant To Data(error in=w500, type=cluster{string, "Data":variant} {"", "Data"=variant}, Variant=w505) -> (data=w503:cluster{string, "Data":variant}, error out=w499:errorcluster)
        n224 = Unbundle(w503) -> (w502:string, "Data"=w501:variant)
        n225 = for {
          tunnel: w506 -> [w513] mode=indexing
          tunnel: w502 -> [w511]
          tunnel: w501 -> [w510]
          shift-right: [w509] -> w496
          shift-left: w499 -> [w508]
          n226 = call "GetViName.vi"("VI*"=w513) -> ("VI Name"=w512:string)  [unwired: 9 in, 1 out]
          n227 = call-poly "QueueManager.vi"("error in"=w508, "Data"=w510, "Event"=w511, "QueueName"=w512) -> ("error out"=w509:errorcluster)  [unwired: 6 in, 1 out]
        }
        n228 = Bundle By Name(cluster=w498, "error"=w496) -> (w497:T1)
      }
      frame "SendToAllPanels" {
        (unwired) cluster{"Event":string, "Data":variant} {"Event"="", "Data"=variant} ("Send")
        # ">> Notes: 发送至所有Page页的所有面板，变体Data的数据结构为包含字符串和变体的簇<<"
        n229 = Unbundle By Name(w519) -> ("Data"=w521:variant)
        n230 = disable-structure shown="\"调用形式如下\"" {
          frame condition #0 {
            n231 = call "UserDefinedQNames.vi"() -> ("All Queues"=w523:T2)  [unwired: 11 in]
            n232 = Unbundle By Name(w523) -> ("CUI Queue"=w522:string)
            n233 = call-poly "QueueManager.vi"("Data"=cluster{"Event":string, "Data":variant} {"Event"="", "Data"=variant} ("Send"), "Event"="SendToAllPanels", "QueueName"=w522) -> ()  [unwired: 7 in, 2 out]
          }
          frame condition #1 (active) {
          }
        }
        n234 = Bundle("SendToAllPanels", "Data"=w521) -> (w518:cluster{string, "Data":variant})  [unwired: 1 in]
        n235 = Bundle By Name(cluster=w519, "Data"=w518) -> (w514:T1)
        n236 = call "Add State(s) to Queue.vi"("State(s) in Front (\"\")"="SendToAll" ("State(s) in Front (\"\")"), "State(s) in (\"\")"=w517) -> ("States Out"=w516:string)  [unwired: 13 in]
      }
    }
  }
  n237 = disable-structure shown="禁用" {
    frame Disabled {
      n238 = Search 1D Array() -> ()  [unwired: 3 in, 1 out]
    }
    frame Enabled {
    }
  }
  n239 = call <vilib>:"Simple Error Handler.vi"("error in (no error)"=w5) -> ()  [unwired: 4 in, 5 out]
  n240 = Unbundle By Name(w10) -> ("Q_Local"=w7:string, "error"=w11:errorcluster)
  n241 = call-poly "QueueManager.vi"("error in (no error)"=w11, "QueeuName"=w7) -> ()  [unwired: 9 in, 1 out]
